vi "Configure BEEP.vi"(0 "VISA resource name":refnum<visa-resource-name>, 5 "BEEP Configuration":i32, 7 "Configuration Query":bool=TRUE, 11 "error in (no error)":errorcluster) -> (4 "VISA resource name out":refnum<visa-resource-name>, 6 "Query Output":string="\r\n", 8 "Error Message":string, 10 "Error Code":i32, 15 "error out":errorcluster)   [LabVIEW 2010, in "VITREK V7X.lvlib"]
doc: "Configures or Query the action of the front panel <b>Beeper</b>.\n\n<b>Note:</b> please refer to the instrument manual for the action of the front panel <b>Beeper</b> specification."
uses:
  VITREK V7X.lvlib
panel:
  # "Yes\n\nNo"
  # "Configures the action of the beeper:\n0 - Off\n1 - Only beep on sequence start and stop\n2 - Only beep on front panel key presses\n3 - Beep for all reasons"
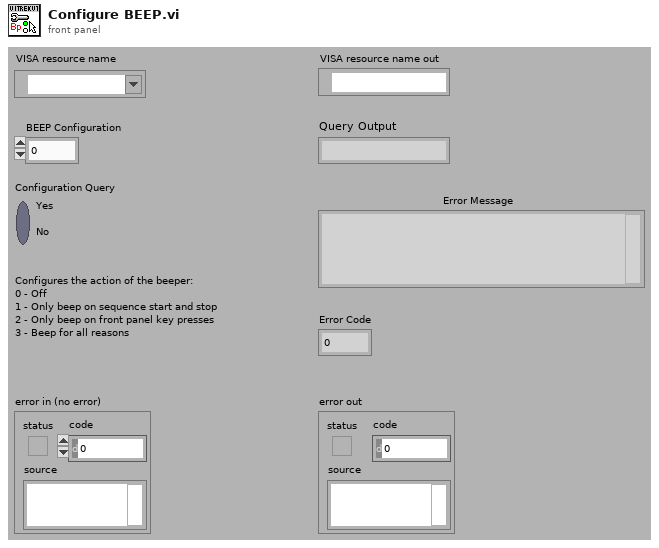
[diagram p1: front panel]
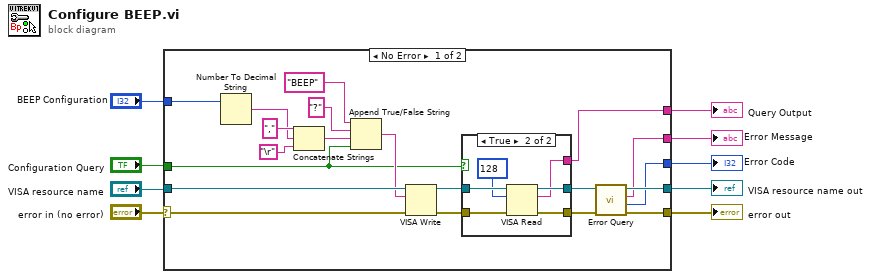
[diagram p0: block diagram]
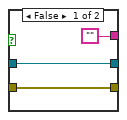
[diagram p2: hidden frame]
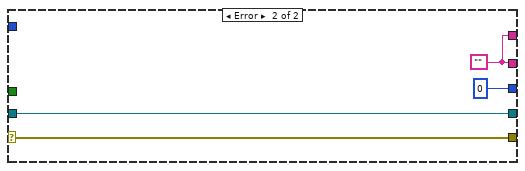
[diagram p3: hidden frame]
diagram:
  n1 = case shown="No Error" "error in (no error)" {
    selector: "error in (no error)" -> [w18 w41]
    tunnel: "VISA resource name" -> [w29 w42]
    tunnel: "Configuration Query" -> [w25 _]
    tunnel: [w23 w40] -> w7
    tunnel: [w20 w42] -> w6
    tunnel: [w19 w41] -> w5
    tunnel: [w13 0 ("Error Code")] -> w3
    tunnel: [w12 w40] -> w2
    tunnel: "BEEP Configuration" -> [w11 _]
    frame No Error {
      n2 = Number To Decimal String(number=w11) -> (decimal integer string=w14:string)  [unwired: 1 in]
      n3 = Concatenate Strings(",", w14, "\r") -> (w15:string)
      n4 = Append True/False String(1:w25, 2:w15, 3:"?", 4:"BEEP" ("command")) -> (0:w27:string)
      n5 = VISA Write(VISA resource name=w29, write buffer=w27, error in (no error)=w18) -> (VISA resource name out=w26:refnum<visa-resource-name>, error out=w24:errorcluster)  [unwired: 1 out]
      n6 = case shown="True" w25 {
        tunnel: w26 -> [w32 w36]
        tunnel: [w32 w34] -> w22
        tunnel: w24 -> [w31 w37]
        tunnel: [w31 w38] -> w21
        tunnel: ["" w33] -> w23
        frame False {
        }
        frame True {
          n7 = VISA Read(VISA resource name=w36, byte count=u32 128, error in (no error)=w37) -> (VISA resource name out=w34:refnum<visa-resource-name>, read buffer=w33:string, error out=w38:errorcluster)  [unwired: 1 out]
        }
      }
      n8 = call "Error Query.vi"("error in (no error)"=w21, "VISA resource name"=w22) -> ("error out"=w19:errorcluster, "Error Code"=w13:i32, "Error Message"=w12:string, "VISA resource name out"=w20:refnum<visa-resource-name>)  [unwired: 6 in]
    }
    frame Error {
      w40 = ""
    }
  }
  "VISA resource name out" <- w6
  "error out" <- w5
  "Query Output" <- w7
  "Error Code" <- w3
  "Error Message" <- w2
